vi "New Entity UI.vi"(10 "Target Name":string, 11 "Project Name":string) -> (0 "Container":string, 1 "Cancelled":bool, 2 "Folder":path, 3 "Entity Name":string, 4 "Library?":bool)   [LabVIEW 2020, in "Conditum-Tools.lvlib" / "Entity Editor.lvclass"]
uses:
  Entity Editor.lvclass
  Entity Editor.lvclass/Entity Editor.ctl
  Conditum-Tools.lvlib
panel:
  in  "Destination Manually Set?":bool
  in  "Destination Folder":path
  in  "Container":i32(listbox)
  out "Message":string
  in  "Cancel":bool
  in  "OK":bool
  in  "Name":string
  # "Select the container in the project to save the entity under:"
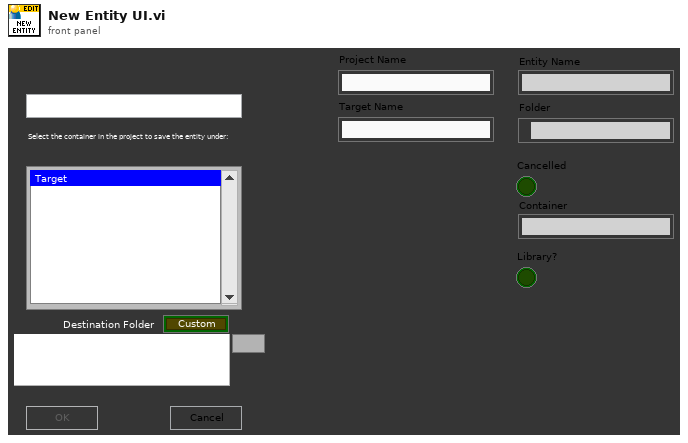
[diagram p1: front panel]
types:
  T1 = enum8{"Enabled", "Disabled", "Disabled and Grayed Out"}
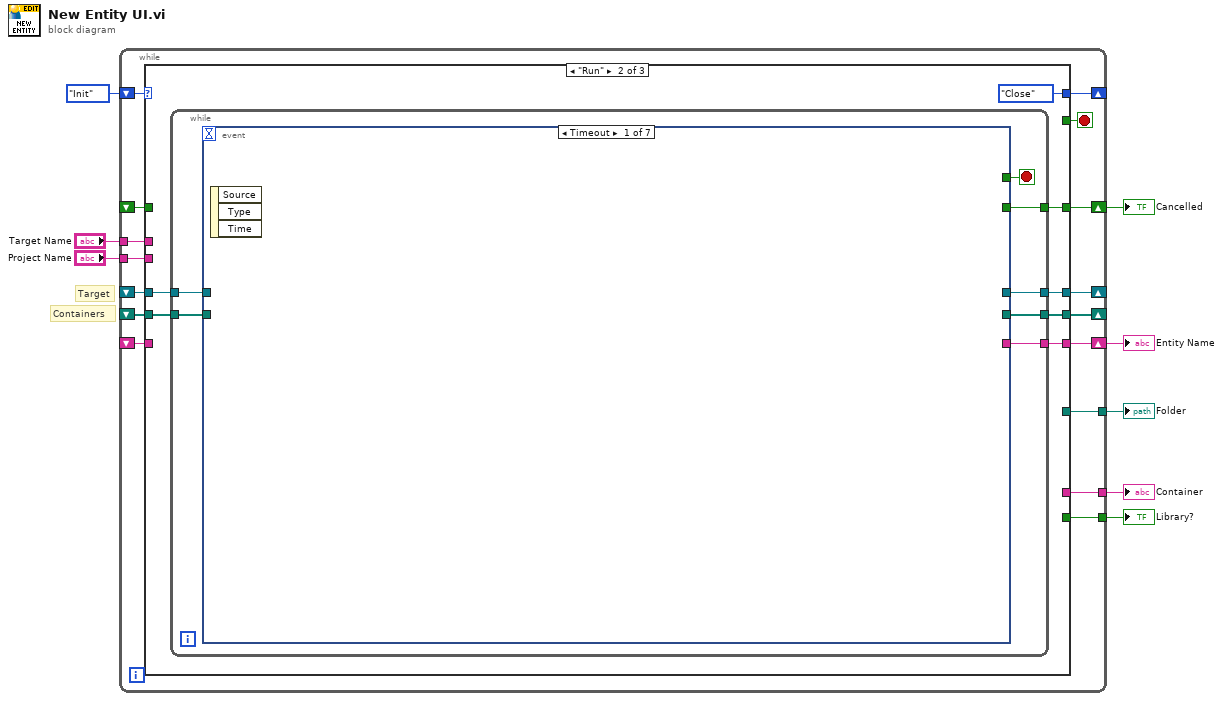
[diagram p0: block diagram]
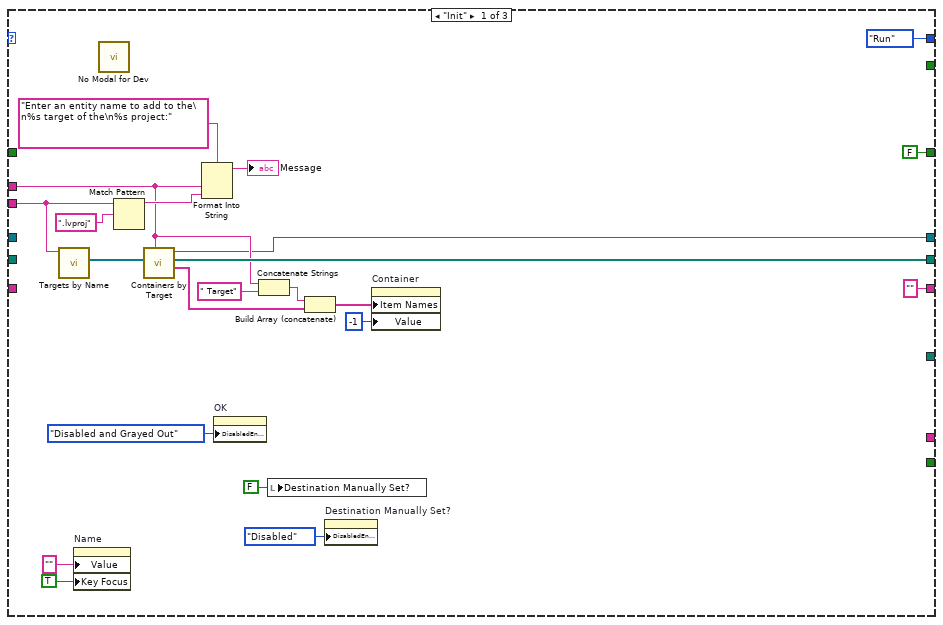
[diagram p2: hidden frame]
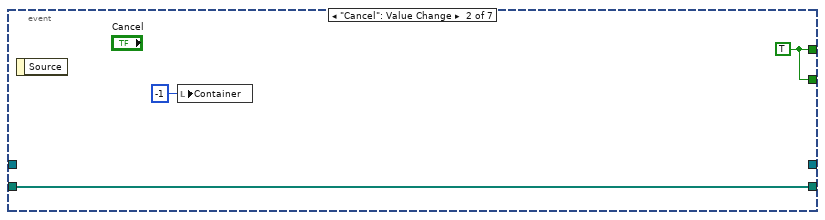
[diagram p3: hidden frame]
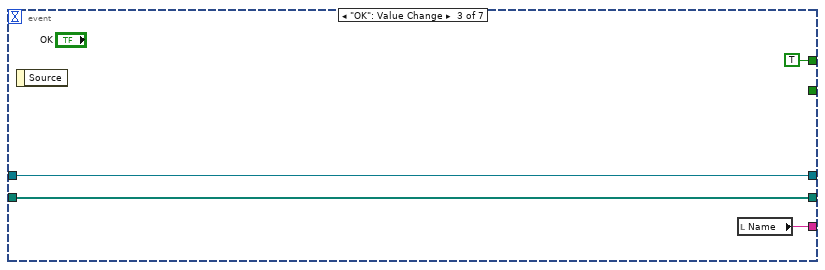
[diagram p4: hidden frame]
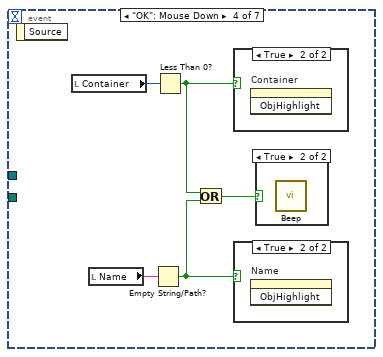
[diagram p5: hidden frame]
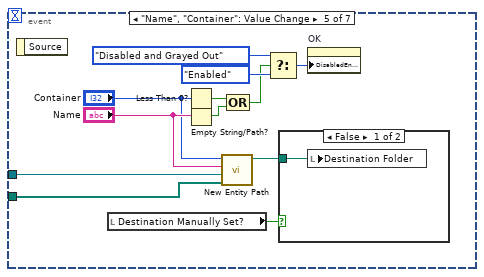
[diagram p9: hidden frame]
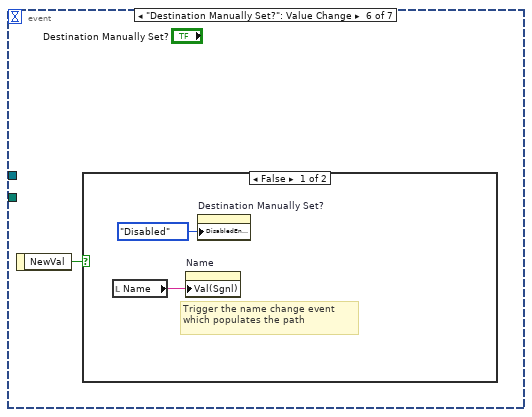
[diagram p11: hidden frame]
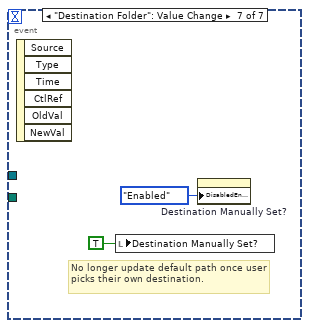
[diagram p13: hidden frame]
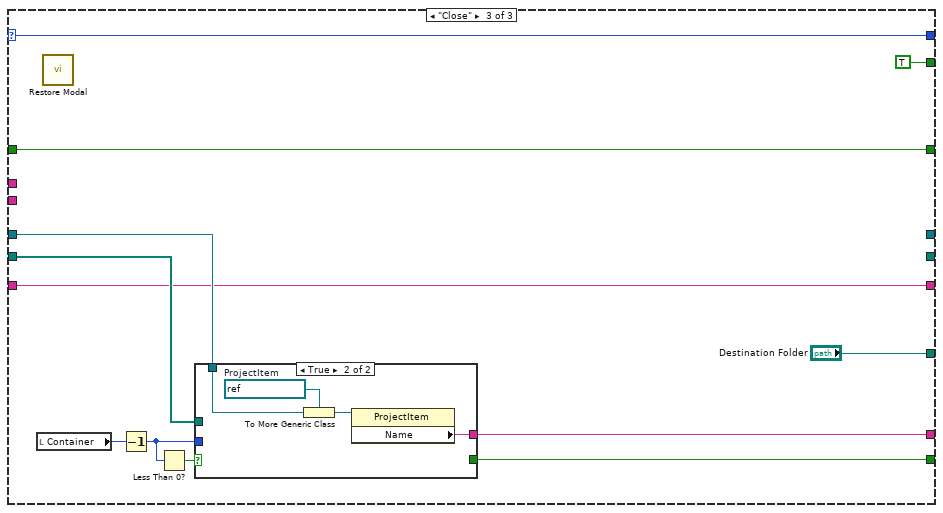
[diagram p14: hidden frame]
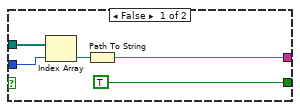
[diagram p15: hidden frame]
diagram:
  # "Containers"
  # "Target"
  n1 = while {
    shift-right: [w23] -> _
    shift-left: enum16{"Init", "Run", "Close"}."Init" ("Basic UI State") -> [w24]
    tunnel: "Project Name" -> [w21]
    shift-right: [w20] -> w6
    shift-left: _ -> [w19]
    tunnel: "Target Name" -> [w18]
    shift-right: [w17] -> w4
    shift-left: _ -> [w16]
    shift-right: [w15] -> _
    shift-left: _ -> [w14]
    tunnel: [w13] -> w3
    shift-right: [w12] -> _
    shift-left: _ -> [w11]
    tunnel: [w10] -> w2
    tunnel: [w9] -> w1
    stop <- w22 stop-if-true
    n2 = case shown="\"Run\"" w24 {
      selector: w24 -> [_ _ w102]
      tunnel: [enum16{"Init", "Run", "Close"}."Run" ("Basic UI State") enum16{"Init", "Run", "Close"}."Close" ("Basic UI State") w102] -> w23
      tunnel: [_ _ TRUE] -> w22
      tunnel: w21 -> [w37 _ _]
      tunnel: [FALSE w52 w100] -> w20
      tunnel: w19 -> [_ _ w100]
      tunnel: w18 -> [w30 _ _]
      tunnel: ["" ("Name") w51 w93] -> w17
      tunnel: w16 -> [_ _ w93]
      tunnel: [w34 w49 _] -> w15
      tunnel: w14 -> [_ w50 w97]
      tunnel: [_ _ w96] -> w13
      tunnel: [w27 w47 _] -> w12
      tunnel: w11 -> [_ w48 w95]
      tunnel: [_ _ "Destination Folder"] -> w10
      tunnel: [_ _ w91] -> w9
      frame "Init" {
        n3 = call "Targets by Name.vi"("Project Name"=w37) -> ("Targets"=w36:refnum<vi>[])  [unwired: 9 in, 1 out]
        n4 = property on="Name" class="Str"("Value"="" ("Name"), "Key Focus"=TRUE) -> ()  [unwired: 2 in, 2 out]
        n5 = call "No Modal for Dev.vi"() -> ()  [unwired: 12 in]
        n6 = Match Pattern(string=w37, regular expression=".lvproj") -> (before substring=w42:string)  [unwired: 1 in, 3 out]
        n7 = call "Containers by Target.vi"("Target Name"=w30, "Targets"=w36) -> ("Container Names"=w35:string[], "Container Paths"=w34:path[], "Target"=w27:refnum<vi>)  [unwired: 7 in]
        n8 = Format Into String(format string="Enter an entity name to add to the\n%s target of the\n%s project:" ("Message"), w30, w42) -> (resulting string=→"Message":string)  [unwired: 2 in, 1 out]
        n9 = property on="OK" class="Bool"("DisabledEnum"=T1."Disabled and Grayed Out" ("Disabled")) -> ()  [unwired: 2 in, 2 out]
        n10 = Concatenate Strings(w30, " Target" ("string")) -> (w29:string)
        n11 = local write "Destination Manually Set?"(FALSE ("Destination Manually Set?")) -> ()
        n12 = Build Array (concatenate)(w29, w35) -> (w31:string[])
        n13 = property on="Destination Manually Set?" class="Bool (strict)"("DisabledEnum"=T1."Disabled" ("Disabled")) -> ()  [unwired: 2 in, 2 out]
        n14 = property on="Container" class="LstBox (strict)"("Item Names"=w31, "Value"=-1 ("Container")) -> ()  [unwired: 2 in, 2 out]
      }
      frame "Run" {
        n15 = while {
          tunnel: [w59] -> w52
          tunnel: [w58] -> w51
          tunnel: w50 -> [w57]
          tunnel: [w56] -> w49
          tunnel: w48 -> [w55]
          tunnel: [w54] -> w47
          stop <- w60 stop-if-true
          n16 = event shown="[0] Timeout" {
            selector: _ -> [_ _ _ _ _ _ _]
            dyn-events: _ -> [_ _ _ _ _ _ _]
            timeout: _ -> [_ _ _ _ _ _ _]
            tunnel: [_ w63 TRUE _ _ _ _] -> w60
            tunnel: [_ w63 _ _ _ _ _] -> w59
            tunnel: [_ _ w65 _ _ _ _] -> w58
            tunnel: w57 -> [_ w62 w66 _ w77 _ _]
            tunnel: [_ w62 w66 _ _ _ _] -> w56
            tunnel: w55 -> [_ _ w64 _ w78 _ _]
            tunnel: [_ _ w64 _ _ _ _] -> w54
            event Timeout {
              n17 = event-data() -> ()  [unwired: 1 in, 3 out]
            }
            event "Cancel": Value Change {
              w63 = TRUE
              n18 = event-data() -> ()  [unwired: 1 in, 1 out]
              n19 = local write "Container"(-1 ("Container")) -> ()
            }
            event "OK": Value Change {
              n20 = event-data() -> ()  [unwired: 1 in, 1 out]
              n21 = local read "Name"() -> (w65:string)
            }
            event "OK": Mouse Down {
              n22 = event-data() -> ()  [unwired: 1 in, 1 out]
              n23 = local read "Container"() -> (w72:i32)
              n24 = local read "Name"() -> (w71:string)
              n25 = Empty String/Path?(string/path=w71) -> (empty?=w69:bool)
              n26 = Less Than 0?(x=w72) -> (x < 0?=w70:bool)
              n27 = Or(x=w70, y=w69) -> (x .or. y?=w68:bool)
              n28 = case shown="True" w70 {
                frame False {
                }
                frame True {
                  n29 = invoke on="Container" class="LstBox (strict)" method="ObjHighlight"() -> ()  [unwired: 3 in, 3 out]
                }
              }
              n30 = case shown="True" w69 {
                frame False {
                }
                frame True {
                  n31 = invoke on="Name" class="Str" method="ObjHighlight"() -> ()  [unwired: 3 in, 3 out]
                }
              }
              n32 = case shown="True" w68 {
                frame False {
                }
                frame True {
                  n33 = call <vilib>:"Beep.vi"() -> ()  [unwired: 12 in]
                }
              }
            }
            event "Name", "Container": Value Change {
              n34 = event-data() -> ()  [unwired: 1 in, 1 out]
              n35 = local read "Destination Manually Set?"() -> (w73:bool)
              n36 = Less Than 0?(x="Container") -> (x < 0?=w81:bool)
              n37 = Empty String/Path?(string/path="Name") -> (empty?=w80:bool)
              n38 = call "New Entity Path.vi"("Container Paths"=w77, "Target"=w78, "Entity Name"="Name", "Container Index"="Container") -> ("Default Entity Folder"=w74:path)  [unwired: 7 in]
              n39 = Compound Arithmetic op=OR(w81, w80) -> (w79:bool)
              n40 = Select(t=T1."Disabled and Grayed Out", s=w79, f=T1."Enabled" ("Disabled")) -> (s? t:f=w82:T1)
              n41 = case shown="False" w73 {
                tunnel: w74 -> [w85 _]
                frame False {
                  n42 = local write "Destination Folder"(w85) -> ()
                }
                frame True {
                }
              }
              n43 = property on="OK" class="Bool"("DisabledEnum"=w82) -> ()  [unwired: 2 in, 2 out]
            }
            event "Destination Manually Set?": Value Change {
              n44 = event-data() -> ("NewVal"=w86:bool)  [unwired: 1 in]
              n45 = case shown="False" w86 {
                frame False {
                  # "Trigger the name change event which populates the path"
                  n46 = local read "Name"() -> (w87:string)
                  n47 = property on="Name" class="Str"("Val(Sgnl)"=w87) -> ()  [unwired: 2 in, 2 out]
                  n48 = property on="Destination Manually Set?" class="Bool (strict)"("DisabledEnum"=T1."Disabled" ("Disabled")) -> ()  [unwired: 2 in, 2 out]
                }
                frame True {
                }
              }
            }
            event "Destination Folder": Value Change {
              # "No longer update default path once user picks their own destination."
              n49 = event-data() -> ()  [unwired: 1 in, 6 out]
              n50 = local write "Destination Manually Set?"(TRUE ("Destination Manually Set?")) -> ()
              n51 = property on="Destination Manually Set?" class="Bool (strict)"("DisabledEnum"=T1."Enabled" ("Disabled")) -> ()  [unwired: 2 in, 2 out]
            }
          }
        }
      }
      frame "Close" {
        n52 = local read "Container"() -> (w94:i32)
        n53 = call "Restore Modal.vi"() -> ()  [unwired: 12 in]
        n54 = Decrement(x=w94) -> (x-1=w98:i32)
        n55 = Less Than 0?(x=w98) -> (x < 0?=w99:bool)
        n56 = case shown="True" w99 {
          tunnel: w98 -> [w106 _]
          tunnel: w97 -> [w107 _]
          tunnel: [w104 w108] -> w96
          tunnel: w95 -> [_ w111]
          tunnel: [TRUE _] -> w91
          frame False {
            n57 = Index Array(array=w107, index=w106) -> (element=w105:path)
            n58 = Path To String(path=w105) -> (string=w104:string)
          }
          frame True {
            w110 = refnum<vi> refnum  # ProjectItem
            n59 = To More Generic Class(target class=w110, reference=w111) -> (generic class reference=w109:refnum<vi>)
            n60 = property class="ProjectItem"(reference=w109) -> ("Name"=w108:string)  [unwired: 1 in, 2 out]
          }
        }
      }
    }
  }
  "Cancelled" <- w6
  "Entity Name" <- w4
  "Container" <- w3
  "Folder" <- w2
  "Library?" <- w1
